vi "BuildMenuItem.vi"(8 "error":errorcluster, 10 "ItemTag":string, 11 "Menu":refnum<class "Menu.lvclass">) -> (0 "error out":errorcluster, 3 "Menu out":refnum<class "Menu.lvclass">)   [LabVIEW 2021, in "Menu.lvlib" / "Menu.lvclass"]
uses:
  Menu.lvclass
  Menu.lvclass/Menu.ctl
  Picture2D/src/Picture/Image.lvclass
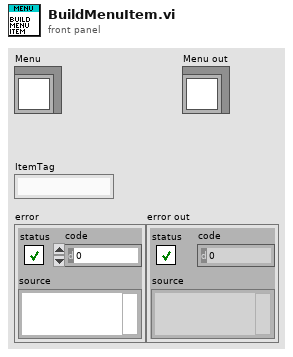
[diagram p1: front panel]
types:
  T1 = typedef "LVMenuShortCut.ctl" = cluster{"include Shift key?":bool, "include Ctrl key?":bool, "shortcut key":string}
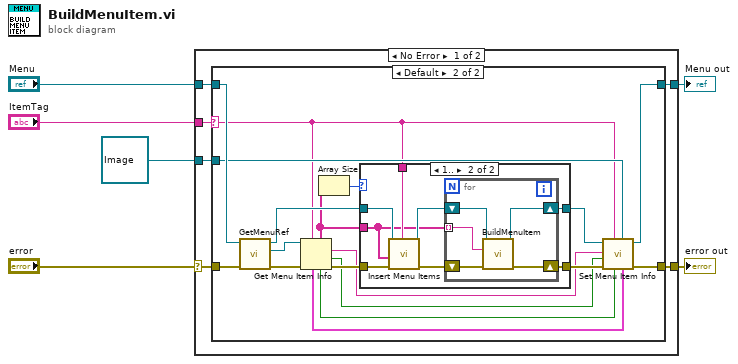
[diagram p0: block diagram]
diagram:
  n1 = case shown="No Error" "error" {
    selector: "error" -> [w12 w49]
    tunnel: [w8 w49] -> w5
    tunnel: [w9 w48] -> w3
    tunnel: "Menu" -> [w11 w48]
    tunnel: "ItemTag" -> [w10 _]
    tunnel: refnum<class "Image.lvclass"> refnum ("Picture") -> [w7 _]
    frame No Error {
      n2 = case shown="Default" w10 {
        selector: w10 -> [_ w15]
        tunnel: w12 -> [w13 w32]
        tunnel: w11 -> [w14 w31]
        tunnel: [w14 w20] -> w9
        tunnel: [w13 w19] -> w8
        tunnel: w7 -> [_ w18]
        frame "" {
        }
        frame Default {
          n3 = call "GetMenuRef.vi"("error in (no error)"=w32, "Menu in"=w31) -> ("error out"=w29:errorcluster, "RTMMenuReference"=w30:refnum<k9>, "Menu out"=w27:refnum<class "Menu.lvclass">)  [unwired: 7 in]
          n4 = Get Menu Item Info(7:w15, 8:w29, 11:w30) -> (0:w28:errorcluster, 1:w23:bool, 2:w22:string, 4:w24:bool, 5:w16:string[], 6:w25:T1)  [unwired: 1 out]
          n5 = Array Size(array=w16) -> (size(s)=w17:i32)
          n6 = case shown="1.." w17 {
            tunnel: w28 -> [w33 w39]
            tunnel: w16 -> [_ w35]
            tunnel: w27 -> [w34 w37]
            tunnel: [w33 w42] -> w26
            tunnel: [w34 w41] -> w21
            tunnel: w15 -> [_ w36]
            frame ..0 {
            }
            frame 1.. {
              n7 = call "Insert Menu Items.vi"("menu tag"=w36, "error in (no error)"=w39, "item tags"=w35, "Menu in"=w37) -> ("error out"=w40:errorcluster, "Menu out"=w38:refnum<class "Menu.lvclass">)  [unwired: 5 in, 1 out]
              n8 = for {
                shift-right: [w46] -> w42
                shift-left: w40 -> [w47]
                tunnel: w35 -> [w45] mode=indexing
                shift-right: [w43] -> w41
                shift-left: w38 -> [w44]
                n9 = call "BuildMenuItem.vi"("error"=w47, "ItemTag"=w45, "Menu"=w44) -> ("error out"=w46:errorcluster, "Menu out"=w43:refnum<class "Menu.lvclass">)  [unwired: 7 in]
              }
            }
          }
          n10 = call "Set Menu Item Info.vi"("short cut"=w25, "Picture"=w18, "checked"=w24, "item tag"=w15, "error in (no error)"=w26, "enabled"=w23, "item name"=w22, "Menu in"=w21) -> ("error out"=w19:errorcluster, "Menu out"=w20:refnum<class "Menu.lvclass">)  [unwired: 2 in]
        }
      }
    }
    frame Error {
    }
  }
  "error out" <- w5
  "Menu out" <- w3
